vi "stepper driver -- wrapper.vi"(4 "motor selector":T1=enum."--", 6 "Instrument Address":refnum<visa-resource-name>="ASRL2::INSTR", 7 "stepper driver action":T3, 10 "speed IN":dbl, 11 "number IN":dbl format="%#_13g") -> (1 "stepper motor state OUT":T2, 2 "speed OUT":dbl, 3 "number OUT":dbl)   [LabVIEW 2020]
uses:
  stepper driver action.ctl
  stepper motor state.ctl
  motor type.ctl
panel:
  out "reference out":refnum<vi>
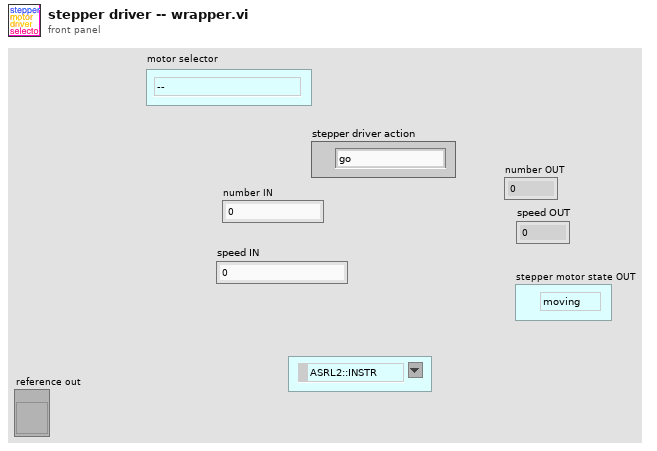
[diagram p1: front panel]
types:
  T1 = typedef "motor type.ctl" = enum16{"IMS", "arduino C&A", "BLM", "--"}
  T2 = typedef "stepper motor state.ctl" = enum16{"moving", "stopped"}
  T3 = typedef "stepper driver action.ctl" = enum16{"go", "void", "stop", "check", "init", "sync", "set", "set speed", "--check status", "--check value", "--handshake"}
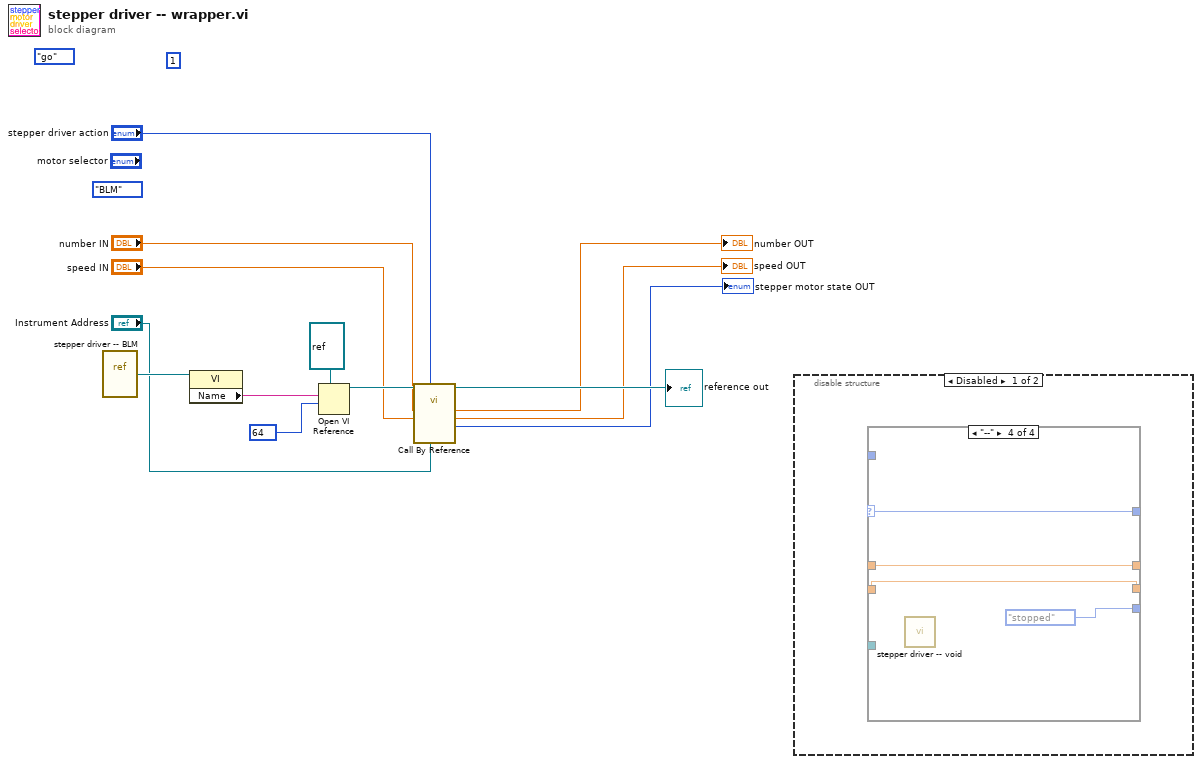
[diagram p0: block diagram]
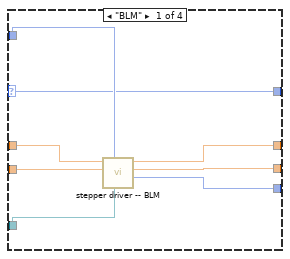
[diagram p2: hidden frame]
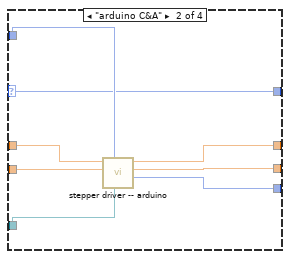
[diagram p3: hidden frame]
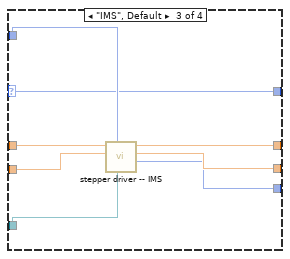
[diagram p4: hidden frame]
diagram:
  (unwired) stepper_driver_action."go" ("stepper driver action")
  (unwired) motor_type."BLM" ("motor selector")
  (unwired) 1
  n1 = vi-ref "stepper driver -- BLM.vi"() -> (w8:refnum<vi>)
  n2 = property class="VI"(reference=w8) -> ("Name"=w12:string)  [unwired: 1 in, 2 out]
  n3 = Open VI Reference(type specifier VI Refnum (for type only)=refnum<vi> refnum, vi path=w12, options=64) -> (vi reference=w9:refnum<vi>)  [unwired: 3 in, 1 out]
  n4 = call-by-ref "?"(reference=w9, "Instrument Address"="Instrument Address", "stepper driver action"="stepper driver action", "speed IN"="speed IN", "number"="number IN") -> (reference out=→"reference out":refnum<vi>, "stepper motor state OUT"=→"stepper motor state OUT":T2, "speed"=→"speed OUT":dbl, "number out"=→"number OUT":dbl)  [unwired: 6 in, 1 out]
  n5 = disable-structure shown="Disabled" {
    frame Disabled {
      n6 = case shown="\"--\"" {
        selector: _ -> [w14 w22 w30 w38]
        tunnel: _ -> [w21 w29 w37 _]
        tunnel: [w20 w28 w36 w40] -> _
        tunnel: [w19 w27 w35 stepper_motor_state."stopped" ("stepper motor state OUT")] -> _
        tunnel: [w18 w26 w34 w41] -> _
        tunnel: _ -> [w17 w25 w33 w41]
        tunnel: _ -> [w16 w24 w32 w40]
        tunnel: _ -> [w15 w23 w31 _]
        tunnel: [w14 w22 w30 w38] -> _
        frame "BLM" {
          n7 = call "stepper driver -- BLM.vi"("Instrument Address"=w15, "stepper driver action"=w21, "speed IN"=w16, "number"=w17) -> ("stepper motor state OUT"=w19:T2, "speed"=w20:dbl, "number out"=w18:dbl)  [unwired: 5 in]
        }
        frame "arduino C&A" {
          n8 = call "stepper driver -- arduino.vi"("Instrument Address"=w23, "stepper driver action"=w29, "speed IN"=w24, "number"=w25) -> ("stepper motor state OUT"=w27:T2, "speed"=w28:dbl, "number out"=w26:dbl)  [unwired: 5 in]
        }
        frame "IMS", Default {
          n9 = call "stepper driver -- IMS.vi"("Instrument Address"=w31, "stepper driver action"=w37, "speed IN"=w32, "number"=w33) -> ("stepper motor state OUT"=w35:T2, "speed"=w36:dbl, "number out"=w34:dbl)  [unwired: 5 in]
        }
        frame "--" {
          n10 = call "stepper driver -- void.vi"() -> ()  [unwired: 9 in, 3 out]
        }
      }
    }
    frame Enabled {
    }
  }
